vi "Omniax_mDrive_Zonly_2017APXNoBK_202107bk.vi"() -> ()   [LabVIEW 2015]
uses:
  <vilib>/Utility/file.llb/Read From Spreadsheet File (I64).vi
  <vilib>/Utility/file.llb/Read From Spreadsheet File (string).vi
  <userlib>/caLab/Private/Put_DBL_PV.vi
  <vilib>/Instr/_visa.llb/VISA Configure Serial Port (Instr).vi
  <userlib>/caLab/Private/Put_DBL-1D_PV-1D.vi
  <userlib>/caLab/Private/Get_PV.vi
  <userlib>/caLab/Private/Put_I16-1D_PV-1D.vi
  <userlib>/caLab/Private/Get_PV-1D.vi
  <vilib>/Utility/file.llb/Write To Spreadsheet File (I64).vi
panel:
  out "Status Message 2":string="HP cell pressure too high! or "
  out "APX:MZ_STOP":bool
  out "inside IV5?":bool
  out "APX:MZ_LIM-":bool
  out "inside PRP?":bool
  out "error out 2":errorcluster caption="error out"
  out "APX:MZ_CHK":u32
  out "APX:MZ_STAT":u32
  out "retracted":bool
  out "facingup":bool
  out "gatevalve":bool
  in  "Local":bool
  out "unsigned 8bit integer":u8
  out "SES is not busy":bool
  out "EPICS RQs":dbl[][](array[numeric])
  out "Status":bool
  in  "Pressure Overide":bool
  in  "Crash Override":bool
  in  "Is the gatevalve opened?\nAPX:MZ_CHK0":bool
  in  "Is the sample facinng up?\nAPX:MZ_CHK1":bool
  in  "Is the source retracted?\nAPX:MZ_CHK2":bool
  out "APX:MZ_MVG":bool
  out "inside HPC?":bool
  out "HPC01<0.001?":bool
  out "APX:V5 opened?":bool
  out "Isolated from GND?":bool
  out "APX:MZ_LIM+":bool
  out "APX:MZ_RDY":bool
  in  "APX:MZ_RQ":dbl=10.0 min=10.0 max=60.0 step=0.1 format="%_6g"
  in  "APX:MZ_VLC_RQ":dbl=0.40000000000000013 min=0.1 max=0.61 step=0.1
  out "Z Velocity SP step/sec":i32=102400 min=1 max=153600
  out "Z Step SP":i32=-20000 min=0 max=102400000 step=500
  out "Z Step PV":i32 max=2000
  out "Dev1AI0 Voltage":dbl
  out "Z max step":i32
  in  "V5 position 15360000":i32
  out "APX:MZ_VLC_PV":dbl format="%.3f"
  out "Presets":i32[][](array[numeric])
  in  "stop":bool
  in  "Tab Control 3":enum32{"Console", "Reset", "Bypass"}(tab)
  out "APX:MZ status":string="Cancel"
  out "Status Message":string="HP cell pressure too high! or "
  in  "Reset Z Position mm":dbl
  out "Reset Z Motor Steps":i32
  in  "Reset":bool
  out "Z Position MV mm":dbl
  in  "Clear ZY":bool
  out "R Backlash steps/sec":i32
  out "R Backlash":i32
  out "R Holding Current %":i32
  out "R Run Current %":i32
  out "R offset deg":dbl
  out "R deg/rev":dbl
  out "R steps/rev":u32
  out "R velocity PV step/sec":i32
  out "Z COM PORT":refnum<visa-resource-name>="COM5"
  out "Z Backlash steps/sec":i32
  out "Z Backlash":i32
  out "Z Holding Current %":i32
  out "Z Run Current %":i32
  out "Z offset mm":dbl
  out "Z mm/rev":dbl
  out "Z steps/rev":u32
  out "Z  velocity PV step/sec":i32=102400
  out "Z MINPOS":i32=-94296
  out "Z MAXPOS":i32=-34296
  out "APX:MZ_PV":dbl format="%_5g"
  out "X velocity PV step/sec":i32
  out "X Backlash steps/sec":i32
  out "X Backlash":i32
  out "X Holding Current %":i32
  out "X Run Current %":i32
  out "X offset mm":dbl
  out "X mm/rev":dbl
  out "X steps/rev":u32
  out "Y Backlash steps/sec":i32
  out "Y Backlash":i32
  out "Y Holding Current %":i32
  out "Y Run Current %":i32
  out "Y offset mm":dbl
  out "Y mm/rev":dbl
  out "Y steps/rev":u32
  out "Y velocity PV step/sec":i32
  in  "APX:MZ_STOP_Button":bool
  # "APX:MZ"
  # "v2022.06"
  # "COM14"
  # "Prep to Main checkpoints"
  # "Disable these"
  # "355.7"
  # "20 degree"
  # "290"
  # "60"
  # "355.7"
  # "10"
  # "289"
  # "55"
types:
  T1 = enum16{"Stop", "Reset", "Run Current", "Holding Current", "Accel Rate", "Decel Rate", "Move to Relative Position", "Move to Absolute Position", "Echo Mode", "Print Parameter", "Send String", "Microstep Resolution", "Set Current Position", "Max Velocity"}
  T2 = enum8{"Enabled", "Disabled", "Disabled and Grayed Out"}
  T3 = cluster{"first row[0]":i64, "first row[1]":i64, "first row[2]":i64, "first row[3]":i64, "first row[4]":i64, "first row[5]":i64, "first row[6]":i64, "first row[7]":i64, "first row[8]":i64}
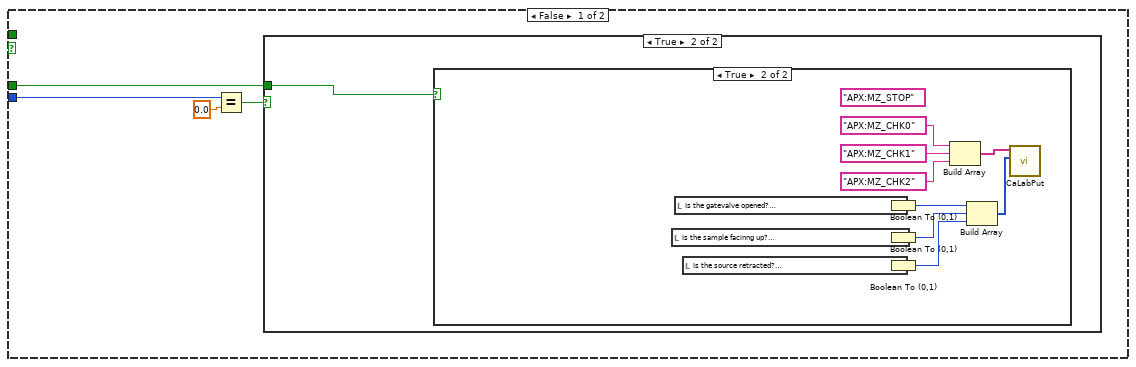
[diagram p3: hidden frame]
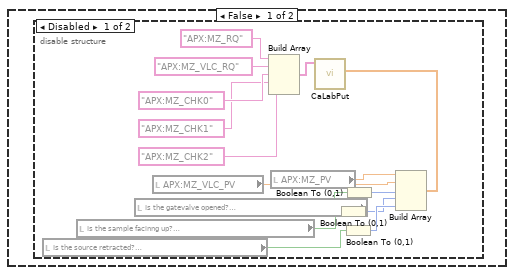
[diagram p5: hidden frame]
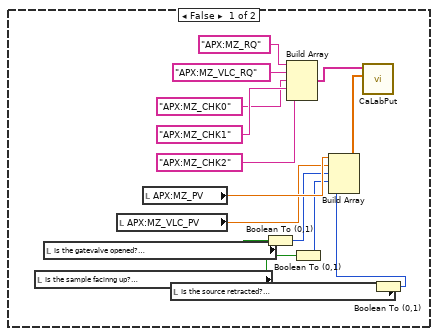
[diagram p7: hidden frame]
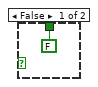
[diagram p10: hidden frame]
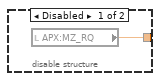
[diagram p12: hidden frame]
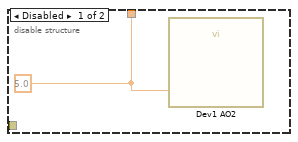
[diagram p14: hidden frame]
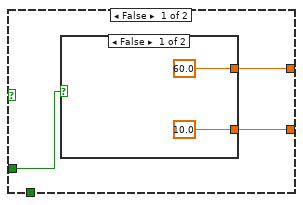
[diagram p16: hidden frame]
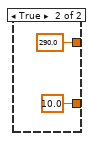
[diagram p17: hidden frame]
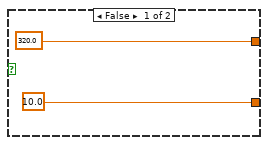
[diagram p18: hidden frame]
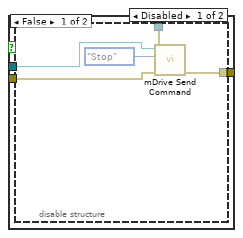
[diagram p19: hidden frame]
diagram:
  w4 = 0 ("dimension size")
  (unwired) 6144000 ("upper limit")
  (unwired) -6144000 ("lower limit")
  n1 = flat-sequence {
    tunnel: [w41] -> w23
    tunnel: [w42] -> w22
    tunnel: w23 -> [w57]
    tunnel: w22 -> [w56]
    tunnel: [w54] -> w2
    tunnel: [w52] -> w1
    tunnel: [w64] -> w27
    tunnel: [w60] -> w26
    tunnel: w2 -> [w61]
    tunnel: w1 -> [w60]
    tunnel: [w71] -> w38
    tunnel: [w73] -> w37
    tunnel: w27 -> [w72]
    tunnel: w26 -> [w74]
    tunnel: w38 -> [w81]
    tunnel: [w80] -> w36
    tunnel: w37 -> [w78]
    tunnel: [w79] -> w35
    tunnel: [w92] -> w34
    tunnel: [w93] -> w33
    tunnel: w36 -> [w91]
    tunnel: w35 -> [w90]
    tunnel: w34 -> [w103]
    tunnel: w33 -> [w102]
    tunnel: [w105] -> w32
    tunnel: [w104] -> w31
    tunnel: [w99] -> w30
    tunnel: [w112] -> w28
    tunnel: [w113] -> w29
    tunnel: w32 -> [w113]
    tunnel: w31 -> [w112]
    tunnel: w30 -> [w110]
    frame #0 {
      n2 = call-poly <userlib>:"CaLabPut.vi"("Value"=1.0, "PV Name"="SES:CalOff_RQ") -> ()  [unwired: 6 in, 4 out]
    }
    frame #1 {
      w49 = refnum<visa-resource-name> "COM14" ("COM PORT")
      w47 = u16 0 items=["None", "XON/XOFF", "RTS/CTS", "XON/XOFF & RTS/CTS", "DTR/DSR", "XON/XOFF & DTR/DSR"] ("flow control (0:none)")
      w46 = u16 10 items=["1.0"=10, "1.5"=15, "2.0"=20] ("stop bits (10: 1 bit)")
      # "Stop bits"
      n3 = call-poly "VISA Configure Serial Port"("VISA resource name"=w49, "timeout (10sec)"=u32 10000, "baud rate (9600)"=u32 9600, "data bits (8)"=u16 8, "parity (0:none)"=enum16{"None", "Odd", "Even", "Mark", "Space"}."None", "stop bits (10: 1 bit)"=w46, "flow control (0:none)"=w47) -> ("VISA resource name out"=w41:refnum<visa-resource-name>, "error out"=w42:errorcluster)  [unwired: 7 in]
      "Z COM PORT" <- w49
    }
    frame #2 {
      n4 = call "mDrive Send Command.vi"("error in (no error)"=w56, "Extra"="EM 2", "Command"=T1."Send String", "VISA resource name"=w57) -> ("error out"=w53:errorcluster, "VISA resource name out"=w55:refnum<visa-resource-name>)  [unwired: 3 in, 1 out]
      n5 = call "mDrive Send Command.vi"("error in (no error)"=w53, "Extra"="PR EE", "Command"=T1."Send String", "VISA resource name"=w55) -> ("error out"=w52:errorcluster, "VISA resource name out"=w54:refnum<visa-resource-name>)  [unwired: 3 in, 1 out]
    }
    frame #3 {
      n6 = Number To Decimal String(number=1000000) -> (decimal integer string=w62:string)  [unwired: 1 in]
      n7 = call "mDrive Send Command.vi"("Extra"=w62, "Command"=T1."Accel Rate", "VISA resource name"=w61) -> ("VISA resource name out"=w67:refnum<visa-resource-name>)  [unwired: 4 in, 2 out]
      n8 = call "mDrive Send Command.vi"("Extra"=w62, "Command"=T1."Decel Rate", "VISA resource name"=w67) -> ("VISA resource name out"=w64:refnum<visa-resource-name>)  [unwired: 4 in, 2 out]
    }
    frame #4 {
      # "Run Current %"
      n9 = property on="Z Run Current %" class="DigNum (strict)"() -> ("Value"=w69:i32)  [unwired: 2 in, 2 out]
      n10 = Number To Decimal String(number=w69) -> (decimal integer string=w70:string)  [unwired: 1 in]
      n11 = call "mDrive Send Command.vi"("error in (no error)"=w74, "Extra"=w70, "Command"=T1."Run Current", "VISA resource name"=w72) -> ("error out"=w73:errorcluster, "VISA resource name out"=w71:refnum<visa-resource-name>)  [unwired: 3 in, 1 out]
    }
    frame #5 {
      # "Holding Current %"
      n12 = property on="Z Run Current %" class="DigNum (strict)"() -> ("Value"=w76:i32)  [unwired: 2 in, 2 out]
      n13 = Number To Decimal String(number=w76) -> (decimal integer string=w77:string)  [unwired: 1 in]
      n14 = call "mDrive Send Command.vi"("error in (no error)"=w78, "Extra"=w77, "Command"=T1."Holding Current", "VISA resource name"=w81) -> ("error out"=w79:errorcluster, "VISA resource name out"=w80:refnum<visa-resource-name>)  [unwired: 3 in, 1 out]
    }
    frame #6 {
      # "Velocity Max"
      n15 = property on="Z Velocity SP step/sec" class="DigNum (strict)"() -> ("Value"=w89:i32)  [unwired: 2 in, 2 out]
      n16 = Number To Decimal String(number=w89) -> (decimal integer string=w88:string)  [unwired: 1 in]
      n17 = call "mDrive Send Command.vi"("error in (no error)"=w90, "Extra"=w88, "Command"=T1."Max Velocity", "VISA resource name"=w91) -> ("error out"=w86:errorcluster, "VISA resource name out"=w96:refnum<visa-resource-name>)  [unwired: 3 in, 1 out]
      n18 = call "mDrive Send Command.vi"("error in (no error)"=w86, "Extra"="VM", "Command"=T1."Print Parameter", "VISA resource name"=w96) -> ("error out"=w93:errorcluster, "read buffer"=w94:string, "VISA resource name out"=w92:refnum<visa-resource-name>)  [unwired: 3 in]
      n19 = Decimal String To Number(string=w94, offset=0) -> (number=w87:i32)  [unwired: 1 in, 1 out]
      n20 = local write "Local"(FALSE ("Remote")) -> ()
      n21 = property on="Z  velocity PV step/sec" class="DigNum (strict)"("Val(Sgnl)"=w87) -> ()  [unwired: 2 in, 2 out]
    }
    frame #7 {
      # "PRINT POSITION"
      n22 = call "mDrive Send Command.vi"("error in (no error)"=w102, "Extra"="P", "Command"=T1."Print Parameter", "VISA resource name"=w103) -> ("error out"=w104:errorcluster, "read buffer"=w101:string, "VISA resource name out"=w105:refnum<visa-resource-name>)  [unwired: 3 in]
      n23 = Decimal String To Number(string=w101, offset=0) -> (number=w99:i32)  [unwired: 1 in, 1 out]
    }
    frame #8 {
      n24 = property on="Z Step SP" class="DigNum (strict)"("Val(Sgnl)"=w110) -> ()  [unwired: 2 in, 2 out]
      n25 = property on="Z Step SP" class="DigNum (strict)"() -> ("Maximum"=w107:dbl)  [unwired: 2 in, 2 out]
      n26 = property on="Z Step SP" class="DigNum (strict)"() -> ("Minimum"=w109:dbl)  [unwired: 2 in, 2 out]
      n27 = To Long Integer(number=w107) -> (32bit integer=w108:i32)
      "Z MAXPOS" <- w108
      n28 = To Long Integer(number=w109) -> (32bit integer=w106:i32)
      "Z MINPOS" <- w106
      n29 = In Range and Coerce(upper limit=w108, x=w110, lower limit=w106) -> (In Range?=w111:bool)  [unwired: 1 out]
      n30 = property on="APX:MZ_LIM+" class="Bool (strict)"("Val(Sgnl)"=w111) -> ()  [unwired: 2 in, 2 out]
    }
  }
  n31 = flat-sequence {
    frame #0 {
      (unwired) 1.0 ("Data Entry Limits:Minimum")
      w117 = -3.0 ("R deg/rev")
      w115 = u32 51200 ("step/rev")
      n32 = To Double Precision Float(number=w115) -> (double precision float=w116:dbl)
      n33 = To Double Precision Float(number=10000 ("Value (Signaling)")) -> (double precision float=w121:dbl)
      n34 = Divide(x=w121, y=w116) -> (x/y=w120:dbl)
      n35 = Multiply(x=w120, y=w117) -> (x*y=w118:dbl)
      n36 = Absolute Value(x=w118) -> ()  [unwired: 1 out]
      "R offset deg" <- 0.0 ("R offset deg")
      "R deg/rev" <- w117
      "R steps/rev" <- w115
    }
  }
  n37 = flat-sequence {
    frame #0 {
      w124 = 0.2 ("Z mm/rev")
      w123 = u32 51200 ("step/rev")
      n38 = To Double Precision Float(number=153600 ("Value (Signaling)")) -> (double precision float=w129:dbl)
      n39 = To Double Precision Float(number=w123) -> (double precision float=w128:dbl)
      n40 = property on="Z Velocity SP step/sec" class="DigNum (strict)"("Val(Sgnl)"=51200 ("Value (Signaling)")) -> ()  [unwired: 2 in, 2 out]
      n41 = property on="Z Velocity SP step/sec" class="DigNum (strict)"("Minimum"=1.0 ("Data Entry Limits:Minimum")) -> ()  [unwired: 2 in, 2 out]
      n42 = Divide(x=w129, y=w128) -> (x/y=w126:dbl)
      n43 = property on="Z Velocity SP step/sec" class="DigNum (strict)"("Maximum"=w129) -> ()  [unwired: 2 in, 2 out]
      n44 = Multiply(x=w126, y=w124) -> (x*y=w127:dbl)
      n45 = property on="APX:MZ_VLC_RQ" class="DigNum (strict)"("Val(Sgnl)"=w127) -> ()  [unwired: 2 in, 2 out]
      "Z offset mm" <- 0.0 ("Z offset mm")
      "Z mm/rev" <- w124
      "Z steps/rev" <- w123
    }
  }
  n46 = disable-structure shown="Disabled" {
    frame Disabled {
      n47 = flat-sequence {
        frame #0 {
          w132 = FALSE ("Value (Signaling)")
          w135 = FALSE ("Value (Signaling)")
          w138 = FALSE ("Value (Signaling)")
          w139 = FALSE ("Value (Signaling)")
          "Z Backlash steps/sec" <- 25600 ("Z Backlash steps/sec")
          "Z Backlash" <- -51200 ("Z Backlash")
          "X Backlash steps/sec" <- 25600 ("Value (Signaling)")
          "X Backlash" <- 10240 ("Backlash2")
          "Y Backlash" <- -10240 ("Backlash2")
          "Y Backlash steps/sec" <- 25600 ("Value (Signaling)")
          "R Backlash steps/sec" <- 6400 ("R Backlash steps/sec")
          "R Backlash" <- -12800 ("R Backlash")
        }
      }
    }
    frame Enabled {
    }
  }
  n48 = flat-sequence {
    frame #0 {
      "Z Holding Current %" <- 20 ("Z Holding Current %")
      "Z Run Current %" <- 40 ("Z Run Current %")
      "X Run Current %" <- 40 ("Run Current %")
      "X Holding Current %" <- 20 ("Holding Current %")
      "Y Run Current %" <- 40 ("Run Current %")
      "Y Holding Current %" <- 20 ("Holding Current %")
      "R Holding Current %" <- 15 ("R Holding Current %")
      "R Run Current %" <- 80 ("R Run Current %")
    }
  }
  n49 = flat-sequence {
    frame #0 {
      (unwired) 0.1 ("Value (Signaling)")
      (unwired) FALSE ("Value (Signaling)")
      (unwired) T2."Disabled and Grayed Out" ("Disabled")
      (unwired) T2."Disabled and Grayed Out" ("Disabled")
      (unwired) 0.1 ("Value (Signaling)")
      (unwired) FALSE ("Value (Signaling)")
      (unwired) 0.1 ("Value (Signaling)")
      (unwired) FALSE ("Value (Signaling)")
      (unwired) 0.1 ("Value (Signaling)")
      (unwired) FALSE ("Value (Signaling)")
    }
  }
  n50 = flat-sequence {
    frame #0 {
      w154 = 0.2 ("MM/rev")
      w156 = u32 51200 ("step/rev")
      (unwired) 1.0 ("Data Entry Limits:Minimum")
      # "a=1000000"
      n51 = To Double Precision Float(number=128000 ("Value (Signaling)")) -> (double precision float=w157:dbl)
      n52 = To Double Precision Float(number=w156) -> (double precision float=w155:dbl)
      n53 = Divide(x=w157, y=w155) -> (x/y=w153:dbl)
      n54 = Multiply(x=w153, y=w154) -> ()  [unwired: 1 out]
      "X offset mm" <- 0.0 ("offset")
      "X steps/rev" <- w156
      "X mm/rev" <- w154
    }
  }
  n55 = flat-sequence {
    frame #0 {
      w161 = 0.2 ("MM/rev")
      w163 = u32 51200 ("step/rev")
      (unwired) 1.0 ("Data Entry Limits:Minimum")
      n56 = To Double Precision Float(number=128000 ("Value (Signaling)")) -> (double precision float=w164:dbl)
      n57 = To Double Precision Float(number=w163) -> (double precision float=w162:dbl)
      n58 = Divide(x=w164, y=w162) -> (x/y=w160:dbl)
      n59 = Multiply(x=w160, y=w161) -> ()  [unwired: 1 out]
      "Y offset mm" <- 0.0 ("offset")
      "Y steps/rev" <- w163
      "Y mm/rev" <- w161
    }
  }
  n60 = property on="Z Step SP" class="DigNum (strict)"("Minimum"=0 ("lower limit")) -> ()  [unwired: 2 in, 2 out]
  n61 = property on="V5 position 15360000" class="DigNum (strict)"("Value"=15360000 ("V5 position 15360000")) -> ()  [unwired: 2 in, 2 out]
  n62 = property on="Z Step SP" class="DigNum (strict)"("Maximum"=102400000 ("upper limit")) -> ()  [unwired: 2 in, 2 out]
  n63 = call-poly <vilib>:"Read From Spreadsheet File.vi"("file path (dialog if empty)"=path "T:/PAR/IMS/POSZ.TXT") -> ("first row"=w18:i64[])  [unwired: 6 in, 4 out]
  n64 = call-poly <vilib>:"Read From Spreadsheet File.vi"("file path (dialog if empty)"=path "T:/PAR/IMS/PRESET.TXT") -> ("all rows"=w10:string[][])  [unwired: 6 in, 4 out]
  n65 = Array To Cluster(array=w18) -> (cluster=w17:T3)
  n66 = Transpose 2D Array(2D array=w10) -> (transposed array=w11:string[][])
  n67 = Unbundle(w17) -> ("first row[2]"=w15:i64)  [unwired: 8 out]
  n68 = Delete From Array(array=w11, index (row)=0) -> (array with subset deleted=w13:string[][])  [unwired: 2 in, 1 out]
  n69 = property on="Reset Z Motor Steps" class="DigNum (strict)"("Val(Sgnl)"=w15) -> ()  [unwired: 2 in, 2 out]
  n70 = Transpose 2D Array(2D array=w13) -> (transposed array=w14:string[][])
  n71 = Decimal String To Number(string=w14) -> (number=w12:i32[][])  [unwired: 2 in, 1 out]
  n72 = Initialize Array(w4, w4, 4 ("dimension size")) -> (w7:i32[][])
  n73 = Build Array (concatenate)(w7, w12) -> (→"Presets":i32[][])
  n74 = while {
    tunnel: w29 -> [w181]
    tunnel: w28 -> [w180]
    tunnel: [w179] -> w21
    tunnel: [w178] -> w20
    tunnel: [w177] -> _
    tunnel: [w176] -> _
    i -> [w168]
    stop <- "stop" stop-if-true
    n75 = flat-sequence {
      frame #0 {
        (unwired) 0
        (unwired) "APX:MZ_STOP"
        n76 = local read "Is the gatevalve opened?\nAPX:MZ_CHK0"() -> (w203:bool)
        n77 = local read "Is the source retracted?\nAPX:MZ_CHK2"() -> (w205:bool)
        n78 = local read "Is the sample facinng up?\nAPX:MZ_CHK1"() -> (w204:bool)
        n79 = local read "SES is not busy"() -> (w189:bool)
        n80 = local read "APX:MZ_LIM+"() -> (w194:bool)
        n81 = local read "APX:MZ_RDY"() -> (w196:bool)
        n82 = local read "APX:MZ_MVG"() -> (w195:bool)
        n83 = local read "APX:MZ_LIM-"() -> (w193:bool)
        n84 = local read "Isolated from GND?"() -> (w192:bool)
        n85 = local read "inside HPC?"() -> (w190:bool)
        n86 = local read "HPC01<0.001?"() -> (w188:bool)
        n87 = local read "APX:V5 opened?"() -> (w191:bool)
        n88 = local read "inside PRP?"() -> (w186:bool)
        n89 = local read "inside IV5?"() -> (w185:bool)
        n90 = local read "Dev1AI0 Voltage"() -> (w183:dbl)
        n91 = Build Array(w196, w195, w194, w193, w192, w191, w186, w185, w190, w189, w188) -> (w187:bool[])
        n92 = Build Array(w203, w204, w205) -> (w206:bool[])
        n93 = Boolean Array To Number(Boolean array=w187) -> (number=w199:u32)
        "APX:MZ_STAT" <- w199
        n94 = Boolean Array To Number(Boolean array=w206) -> (number=w200:u32)
        "APX:MZ_CHK" <- w200
        n95 = Build Array(w200, w199, w183) -> (w197:dbl[])
        n96 = Build Array("APX:MZ_CHK", "APX:MZ_STAT", "SSE:Tsample") -> (w198:string[])
        n97 = call-poly <userlib>:"CaLabPut.vi"("Values"=w197, "PV Names"=w198) -> ()  [unwired: 6 in, 4 out]
      }
    }
    n98 = Quotient & Remainder(x=w168, y=2) -> (x-y*floor(x/y)=w173:i32)  [unwired: 1 out]
    n99 = Greater?(x=w168, y=2.0) -> (0:w169:bool)
    n100 = Equal To 0?(x=w173) -> (x = 0?=w174:bool)
    n101 = case shown="True" w174 {
      tunnel: [FALSE ("Status") TRUE ("Status")] -> w171
      frame False {
      }
      frame True {
      }
    }
    n102 = Not(x="Local") -> (.not. x?=w166:bool)
    n103 = case shown="True" w169 {
      tunnel: w171 -> [_ w239]
      tunnel: w168 -> [w209 _]
      tunnel: w166 -> [w207 w238]
      frame False {
        n104 = Equal?(x=w209, y=0.0) -> (x = y?=w208:bool)
        n105 = case shown="True" w208 {
          tunnel: w207 -> [_ w211]
          frame False {
          }
          frame True {
            n106 = case shown="True" w211 {
              frame False {
                n107 = disable-structure shown="Disabled" {
                  frame Disabled {
                    n108 = local read "Is the source retracted?\nAPX:MZ_CHK2"() -> (w212:bool)
                    n109 = local read "Is the sample facinng up?\nAPX:MZ_CHK1"() -> (w213:bool)
                    n110 = local read "Is the gatevalve opened?\nAPX:MZ_CHK0"() -> (w214:bool)
                    n111 = local read "APX:MZ_VLC_PV"() -> (w221:dbl)
                    n112 = Build Array("APX:MZ_RQ", "APX:MZ_VLC_RQ", "APX:MZ_CHK0", "APX:MZ_CHK1", "APX:MZ_CHK2") -> (w224:string[])
                    n113 = local read "APX:MZ_PV"() -> (w222:dbl)
                    n114 = Boolean To (0,1)(Boolean=w213) -> (0, 1=w215:i16)
                    n115 = Boolean To (0,1)(Boolean=w212) -> (0, 1=w217:i16)
                    n116 = Boolean To (0,1)(Boolean=w214) -> (0, 1=w216:i16)
                    n117 = Build Array(w222, w221, w216, w215, w217) -> (w223:dbl[])
                    n118 = call-poly <userlib>:"CaLabPut.vi"("Values"=w223, "PV Names"=w224) -> ()  [unwired: 6 in, 4 out]
                  }
                  frame Enabled {
                  }
                }
              }
              frame True {
                (unwired) "APX:MZ_STOP"
                n119 = local read "Is the sample facinng up?\nAPX:MZ_CHK1"() -> (w232:bool)
                n120 = local read "Is the gatevalve opened?\nAPX:MZ_CHK0"() -> (w233:bool)
                n121 = local read "Is the source retracted?\nAPX:MZ_CHK2"() -> (w231:bool)
                n122 = Boolean To (0,1)(Boolean=w233) -> (0, 1=w230:i16)
                n123 = Boolean To (0,1)(Boolean=w232) -> (0, 1=w229:i16)
                n124 = Boolean To (0,1)(Boolean=w231) -> (0, 1=w228:i16)
                n125 = Build Array("APX:MZ_CHK0", "APX:MZ_CHK1", "APX:MZ_CHK2") -> (w234:string[])
                n126 = Build Array(w230, w229, w228) -> (w227:i16[])
                n127 = call-poly <userlib>:"CaLabPut.vi"("Values"=w227, "PV Names"=w234) -> ()  [unwired: 6 in, 4 out]
              }
            }
          }
        }
      }
      frame True {
        n128 = case shown="True" w238 {
          frame False {
            n129 = local read "Is the sample facinng up?\nAPX:MZ_CHK1"() -> (w245:bool)
            n130 = local read "Is the gatevalve opened?\nAPX:MZ_CHK0"() -> (w246:bool)
            n131 = local read "APX:MZ_VLC_PV"() -> (w247:dbl)
            n132 = local read "APX:MZ_PV"() -> (w248:dbl)
            n133 = local read "Is the source retracted?\nAPX:MZ_CHK2"() -> (w244:bool)
            n134 = Boolean To (0,1)(Boolean=w246) -> (0, 1=w243:i16)
            n135 = Build Array("APX:MZ_RQ", "APX:MZ_VLC_RQ", "APX:MZ_CHK0", "APX:MZ_CHK1", "APX:MZ_CHK2") -> (w251:string[])
            n136 = Boolean To (0,1)(Boolean=w245) -> (0, 1=w242:i16)
            n137 = Boolean To (0,1)(Boolean=w244) -> (0, 1=w241:i16)
            n138 = Build Array(w248, w247, w243, w242, w241) -> (w240:dbl[])
            n139 = call-poly <userlib>:"CaLabPut.vi"("Values"=w240, "PV Names"=w251) -> ()  [unwired: 6 in, 4 out]
          }
          frame True {
            w273 = 0 ("index (col)")
            n140 = Build Array("APX:MZ_RQ", "APX:MZ_VLC_RQ", "APX:MZ_STOP", "APX:MZ_CHK0", "APX:MZ_CHK1", "APX:MZ_CHK2") -> (w301:string[])
            n141 = call-poly "CaLabGet.vi"("PV Names"=w301) -> ("Value Array (number)"=w272:dbl[][])  [unwired: 8 in, 6 out]
            "EPICS RQs" <- w272
            n142 = Index Array(array=w272, index (row)=0, index (col)=w273) -> (element=w293:dbl)
            n143 = Index Array(array=w272, index (row)=1, index (col)=w273) -> (element=w296:dbl)
            n144 = Index Array(array=w272, index (row)=2, index (col)=w273) -> (element=w285:dbl)
            n145 = Index Array(array=w272, index (row)=3, index (col)=w273) -> (element=w283:dbl)
            n146 = Index Array(array=w272, index (row)=4, index (col)=w273) -> (element=w270:dbl)
            n147 = Index Array(array=w272, index (row)=5, index (col)=w273) -> (element=w267:dbl)
            n148 = To Unsigned Byte Integer(number=w283) -> (unsigned 8bit integer=w282:u8)
            n149 = To Unsigned Byte Integer(number=w270) -> (unsigned 8bit integer=w271:u8)
            n150 = To Unsigned Byte Integer(number=w267) -> (unsigned 8bit integer=w268:u8)
            n151 = To Unsigned Byte Integer(number=w285) -> (unsigned 8bit integer=w265:u8)
            "unsigned 8bit integer" <- w265
            n152 = In Range and Coerce(upper limit=0.6, x=w296, lower limit=0.1) -> (coerced(x)=w289:dbl)  [unwired: 1 out]
            n153 = In Range and Coerce(upper limit=355.7, x=w293, lower limit=10.0) -> (coerced(x)=w290:dbl)  [unwired: 1 out]
            n154 = Number To Boolean Array(number=w282) -> (Boolean array=w276:bool[])
            n155 = Number To Boolean Array(number=w271) -> (Boolean array=w269:bool[])
            n156 = Number To Boolean Array(number=w268) -> (Boolean array=w266:bool[])
            n157 = Index Array(array=w276, index=0) -> (element=w258:bool)
            "gatevalve" <- w258
            n158 = Index Array(array=w269, index=0) -> (element=w259:bool)
            "facingup" <- w259
            n159 = Index Array(array=w266, index=0) -> (element=w260:bool)
            "retracted" <- w260
            n160 = Number To Boolean Array(number=w265) -> (Boolean array=w257:bool[])
            n161 = local write "Is the source retracted?\nAPX:MZ_CHK2"(w260) -> ()
            n162 = local read "APX:MZ_RQ"() -> (w264:dbl)
            n163 = local write "Is the gatevalve opened?\nAPX:MZ_CHK0"(w258) -> ()
            n164 = local read "APX:MZ_VLC_RQ"() -> (w263:dbl)
            n165 = Index Array(array=w257, index=0) -> (element=w255:bool)
            n166 = local write "Is the sample facinng up?\nAPX:MZ_CHK1"(w259) -> ()
            n167 = local write "APX:MZ_STOP"(w255) -> ()
            n168 = Equal?(x=w264, y=w290) -> (x = y?=w262:bool)
            n169 = Equal?(x=w263, y=w289) -> (x = y?=w261:bool)
            n170 = case shown="False" w262 {
              tunnel: w290 -> [w303 _]
              frame False {
                n171 = property on="APX:MZ_RQ" class="DigNum (strict)"("Val(Sgnl)"=w303) -> ()  [unwired: 2 in, 2 out]
              }
              frame True {
              }
            }
            n172 = case shown="False" w261 {
              tunnel: w289 -> [w302 _]
              frame False {
                n173 = property on="APX:MZ_VLC_RQ" class="DigNum (strict)"("Val(Sgnl)"=w302) -> ()  [unwired: 2 in, 2 out]
              }
              frame True {
              }
            }
          }
        }
        "Status" <- w239
      }
    }
    n174 = event shown="[0] Timeout" {
      selector: _ -> [_ _ _ _ _ _]
      dyn-events: _ -> [_ _ _ _ _ _]
      timeout: 100 -> [_ _ _ _ _ _]
      tunnel: w181 -> [w338 _ _ w662 w737 w746]
      tunnel: w180 -> [w339 _ _ w661 w736 w745]
      tunnel: [w353 _ _ w659 w735 _] -> w179
      tunnel: [w352 _ _ w660 w734 _] -> w178
      tunnel: [_ _ _ _ _ w744] -> w177
      tunnel: [_ _ _ _ _ w743] -> w176
      event Timeout {
        n175 = event-data() -> ()  [unwired: 1 in, 2 out]
        n176 = disable-structure shown="Disabled" {
          frame Disabled {
            n177 = property on="Local" class="Bool (strict)"() -> ("Value"=w365:bool)  [unwired: 2 in, 2 out]
            n178 = case shown="True" w365 {
              frame False {
              }
              frame True {
                n179 = disable-structure shown="Enabled" {
                  disable-tunnel: [w368 w369] -> w366
                  frame Disabled {
                    n180 = local read "APX:MZ_RQ"() -> (w368:dbl)
                  }
                  frame Enabled {
                    n181 = property on="APX:MZ_RQ" class="DigNum (strict)"() -> ("Value"=w369:dbl)  [unwired: 2 in, 2 out]
                  }
                }
                n182 = call-poly <userlib>:"CaLabPut.vi"("Value"=w366, "PV Name"="APX:MZ_RQ") -> ()  [unwired: 6 in, 4 out]
              }
            }
          }
          frame Enabled {
          }
        }
        n183 = property on="Is the gatevalve opened?\nAPX:MZ_CHK0" class="Bool (strict)"() -> ("Value"=w324:bool)  [unwired: 2 in, 2 out]
        n184 = property on="Is the sample facinng up?\nAPX:MZ_CHK1" class="Bool (strict)"() -> ("Value"=w325:bool)  [unwired: 2 in, 2 out]
        n185 = property on="Is the source retracted?\nAPX:MZ_CHK2" class="Bool (strict)"() -> ("Value"=w326:bool)  [unwired: 2 in, 2 out]
        n186 = property on="Isolated from GND?" class="Bool (strict)"() -> ("Value"=w343:bool)  [unwired: 2 in, 2 out]
        n187 = property on="Is the source retracted?\nAPX:MZ_CHK2" class="Bool (strict)"() -> ("Value"=w334:bool)  [unwired: 2 in, 2 out]
        n188 = And(x=w325, y=w326) -> (x .and. y?=w323:bool)
        n189 = And(x=w324, y=w323) -> (x .and. y?=w322:bool)
        n190 = flat-sequence {
          tunnel: [w413] -> w335
          frame #0 {
            n191 = case shown="False" "Pressure Overide" {
              tunnel: [w415 TRUE] -> w413
              frame False {
                n192 = call-poly "CaLabGet.vi"("PV Name"="APX:HPC01") -> ("1rst Value (number)"=w430:dbl, "Error out"=w427:errorcluster)  [unwired: 8 in, 5 out]
                n193 = call-poly "CaLabGet.vi"("PV Name"="APX:V5_SOP", "Error in (no error)"=w427) -> ("1rst Value (number)"=w426:dbl, "Error out"=w419:errorcluster)  [unwired: 7 in, 5 out]
                n194 = call-poly "CaLabGet.vi"("PV Name"="SES:BUSY", "Error in (no error)"=w419) -> ("1rst Value (number)"=w418:dbl)  [unwired: 7 in, 6 out]
                n195 = Less?(x=w430, y=0.001) -> (x < y?=w424:bool)
                "HPC01<0.001?" <- w424
                n196 = Equal?(x=w418, y=0.0) -> (x = y?=w414:bool)
                "SES is not busy" <- w414
                n197 = Number To Boolean Array(number=w426) -> (Boolean array=w425:bool[])
                n198 = case shown="True" w424 {
                  tunnel: ["HP cell pressure too high!" w435] -> w423
                  frame False {
                  }
                  frame True {
                    n199 = local read "Status Message"() -> (w435:string)
                  }
                }
                n200 = Index Array(array=w425) -> (element=w421:bool)  [unwired: 1 in]
                "APX:V5 opened?" <- w421
                n201 = case shown="False" w421 {
                  tunnel: ["HP Turbo GV is closed." w433] -> w422
                  frame False {
                  }
                  frame True {
                    n202 = local read "Status Message"() -> (w433:string)
                  }
                }
                n203 = Or(x=w424, y=w421) -> (x .or. y?=w416:bool)
                n204 = Or(x=w416, y=w414) -> (x .or. y?=w415:bool)
                n205 = local write "Status Message"(w423) -> ()
                n206 = local write "Status Message"(w422) -> ()
              }
              frame True {
              }
            }
          }
        }
        n207 = property on="Is the sample facinng up?\nAPX:MZ_CHK1" class="Bool (strict)"() -> ("Value"=w333:bool)  [unwired: 2 in, 2 out]
        n208 = case shown="True" w322 {
          tunnel: [w500 w501] -> w351
          frame False {
            n209 = property on="V5 position 15360000" class="DigNum (strict)"() -> ("Value"=w500:i32)  [unwired: 2 in, 2 out]
          }
          frame True {
            n210 = property on="Z Step SP" class="DigNum (strict)"() -> ("Maximum"=w501:dbl)  [unwired: 2 in, 2 out]
          }
        }
        "Z max step" <- w351
        n211 = local read "APX:MZ_VLC_PV"() -> (w317:dbl)
        n212 = Build Array("APX:MZ_PV" ("PV Name"), "APX:MZ_VLC_PV" ("PV Name")) -> (w314:string[])
        n213 = property on="Is the gatevalve opened?\nAPX:MZ_CHK0" class="Bool (strict)"() -> ("Value"=w340:bool)  [unwired: 2 in, 2 out]
        n214 = And(x=w333, y=w334) -> (x .and. y?=w332:bool)
        n215 = property on="APX:MZ_PV" class="DigNum (strict)"() -> ("Value"=w316:dbl)  [unwired: 2 in, 2 out]
        n216 = Build Array(w316, w317) -> (w315:dbl[])
        n217 = And(x=w340, y=w332) -> (x .and. y?=w346:bool)
        n218 = property on="inside HPC?" class="Bool (strict)"() -> ("Value"=w341:bool)  [unwired: 2 in, 2 out]
        n219 = call-poly <userlib>:"CaLabPut.vi"("Values"=w315, "PV Names"=w314) -> ()  [unwired: 6 in, 4 out]
        n220 = Greater Or Equal?(x=w316, y=320.0) -> (x >= y?=w327:bool)
        n221 = And(x=w343, y=w346) -> (x .and. y?=w321:bool)
        n222 = Greater?(x=w316, y=55.0) -> (0:w347:bool)
        n223 = Greater?(x=w316, y=289.0) -> (0:w331:bool)
        n224 = flat-sequence {
          frame #0 {
            w371 = 5 ("number of samples")
            # "ai16 p0.16"
            # "Crash Sensing"
            n225 = call "Dev1 AI0"("number of samples"=w371) -> ("data"=w376:dynamicdata, "error out"=w370:errorcluster)  [unwired: 16 in, 1 out]
            n226 = call "Convert from Dynamic Data"("Dynamic Data Type"=w376) -> ("Array"=w377:dbl[])  [unwired: 3 in]
            n227 = disable-structure shown="Enabled" {
              disable-tunnel: [w383 5.0 ("data")] -> w382
              disable-tunnel: w370 -> [_ w385]
              frame Disabled {
                w383 = 5.0 ("data")
                n228 = call "Dev1 AO2"("data"=w383) -> ()  [unwired: 17 in, 2 out]
              }
              frame Enabled {
                n229 = call "Dev1 P1.7"("data"=bool[] [TRUE], "error in"=w385) -> ("error out"=→"error out 2":errorcluster)  [unwired: 16 in, 1 out]
              }
            }
            n230 = Add Array Elements(numeric array=w377) -> (sum=w375:dbl)
            n231 = Divide(x=w375, y=w371) -> (x/y=w374:dbl)
            n232 = Absolute Value(x=w374) -> (abs(x)=w378:dbl)
            "Dev1AI0 Voltage" <- w378
            n233 = Multiply(x=w382, y=0.8) -> (x*y=w372:dbl)
            n234 = Greater?(x=w378, y=w372) -> (0:w379:bool)
            n235 = case shown="True" "Crash Override" {
              tunnel: [w388 TRUE] -> w380
              tunnel: w379 -> [w388 _]
              frame False {
              }
              frame True {
              }
            }
            "Isolated from GND?" <- w380
          }
        }
        n236 = case shown="False" w347 {
          tunnel: w343 -> [w447 _]
          tunnel: [w447 w455] -> w336
          tunnel: w321 -> [_ w455]
          tunnel: ["Sample is grounded!" w453] -> w344
          tunnel: w331 -> [_ w454]
          tunnel: w341 -> [_ w452]
          tunnel: w340 -> [_ w451]
          tunnel: w333 -> [_ w450]
          tunnel: [TRUE FALSE] -> w312
          tunnel: [FALSE TRUE] -> w311
          frame False {
            w438 = 0.0 ("element")
            w445 = FALSE ("Open?")
            n237 = Build Array("APX:MZ_CHK0" ("PV Name"), "APX:MZ_CHK1" ("PV Name"), "APX:MZ_CHK2" ("PV Name")) -> (w442:string[])
            n238 = property on="Is the gatevalve opened?\nAPX:MZ_CHK0" class="Bool (strict)"("Value"=w445) -> ()  [unwired: 2 in, 2 out]
            n239 = Build Array(w438, w438, w438) -> (w437:dbl[])
            n240 = property on="Is the source retracted?\nAPX:MZ_CHK2" class="Bool (strict)"("Value"=w445) -> ()  [unwired: 2 in, 2 out]
            n241 = property on="Is the sample facinng up?\nAPX:MZ_CHK1" class="Bool (strict)"("Value"=w445) -> ()  [unwired: 2 in, 2 out]
            n242 = call-poly <userlib>:"CaLabPut.vi"("Values"=w437, "PV Names"=w442) -> ()  [unwired: 6 in, 4 out]
          }
          frame True {
            n243 = case shown="False" w454 {
              tunnel: [w457 "Be careful, the sample enters into the HP cell!"] -> w453
              tunnel: w452 -> [_ _]
              tunnel: w451 -> [w462 _]
              tunnel: w450 -> [w461 _]
              frame False {
                w458 = "\r"
                w457 = "Is the gate valve opened? Is the sample facing up?  Is the lamp heater retracted?"
                n244 = disable-structure shown="Disabled" {
                  disable-tunnel: w462 -> [w467 _]
                  disable-tunnel: w461 -> [w466 _]
                  disable-tunnel: [w465 _] -> w460
                  disable-tunnel: [w464 _] -> w459
                  frame Disabled {
                    n245 = case shown="True" w467 {
                      tunnel: ["Is the sample facing up?" ""] -> w465
                      frame False {
                      }
                      frame True {
                      }
                    }
                    n246 = case shown="True" w466 {
                      tunnel: ["Is the gate valve opened?" ""] -> w464
                      frame False {
                      }
                      frame True {
                      }
                    }
                  }
                  frame Enabled {
                  }
                }
                n247 = property on="inside HPC?" class="Bool (strict)"("Value"=FALSE ("inside HPC?")) -> ()  [unwired: 2 in, 2 out]
                n248 = Concatenate Strings(w460, w458, w459, w458, w457) -> (w456:string)
                n249 = local write "Status Message"(w456) -> ()
              }
              frame True {
                w473 = 0.1 ("APX:MZ_VLC_RQ")
                n250 = property on="APX:MZ_VLC_RQ" class="DigNum (strict)"("Value"=w473) -> ()  [unwired: 2 in, 2 out]
                n251 = property on="inside HPC?" class="Bool (strict)"("Value"=TRUE ("inside HPC?")) -> ()  [unwired: 2 in, 2 out]
                n252 = call-poly <userlib>:"CaLabPut.vi"("Value"=w473, "PV Name"="APX:MZ_VLC_RQ") -> ()  [unwired: 6 in, 4 out]
                n253 = local write "Status Message 2"("Sample is touching HPC!") -> ()
              }
            }
          }
        }
        n254 = local write "inside PRP?"(w312) -> ()
        n255 = local write "inside IV5?"(w311) -> ()
        n256 = case shown="True" w335 {
          tunnel: w339 -> [w406 w411]
          tunnel: [w405 w411] -> w337
          tunnel: w338 -> [w404 _]
          frame False {
            n257 = disable-structure shown="Disabled" {
              disable-tunnel: w406 -> [w409 _]
              disable-tunnel: [w408 _] -> w405
              disable-tunnel: w404 -> [w407 _]
              frame Disabled {
                n258 = call "mDrive Send Command.vi"("error in (no error)"=w409, "Command"=T1."Stop", "VISA resource name"=w407) -> ("error out"=w408:errorcluster)  [unwired: 4 in, 2 out]
              }
              frame Enabled {
              }
            }
          }
          frame True {
          }
        }
        n259 = Or(x=w335, y=w336) -> (x .or. y?=w320:bool)
        n260 = property on="Isolated from GND?" class="Bool (strict)"() -> ("Value"=w319:bool)  [unwired: 2 in, 2 out]
        n261 = case shown="True" w331 {
          tunnel: [w392 w399] -> w330
          tunnel: [w391 w398] -> w329
          tunnel: w327 -> [_ w397]
          tunnel: w321 -> [w390 _]
          frame False {
            n262 = case shown="False" w390 {
              tunnel: [60.0 ("Data Entry Limits:Maximum") 290.0 ("Data Entry Limits:Maximum")] -> w392
              tunnel: [10.0 ("Data Entry Limits:Minimum") 10.0 ("Data Entry Limits:Minimum")] -> w391
              frame False {
              }
              frame True {
              }
            }
          }
          frame True {
            n263 = case shown="True" w397 {
              tunnel: [320.0 ("Data Entry Limits:Maximum") 355.7 ("Data Entry Limits:Maximum")] -> w399
              tunnel: [10.0 ("Data Entry Limits:Minimum") 290.0 ("Data Entry Limits:Minimum")] -> w398
              frame False {
              }
              frame True {
              }
            }
          }
        }
        n264 = And(x=w320, y=w319) -> (x .and. y?=w308:bool)
        n265 = local read "APX:MZ_STOP"() -> (w310:bool)
        n266 = Equal?(x=w310, y=FALSE) -> (x = y?=w307:bool)
        n267 = And(x=w308, y=w307) -> (x .and. y?=w306:bool)
        n268 = case shown="False" w306 {
          tunnel: w338 -> [w484 w497]
          tunnel: [w483 w497] -> w350
          tunnel: [w481 w494] -> w349
          tunnel: w344 -> [w480 _]
          tunnel: w343 -> [w479 _]
          tunnel: [w478 w496] -> w342
          tunnel: w341 -> [_ w495]
          tunnel: w337 -> [w477 w494]
          frame False {
            n269 = case shown="True" w479 {
              tunnel: w480 -> [w485 w487]
              tunnel: [w485 "Be careful!"] -> w478
              frame False {
              }
              frame True {
                n270 = disable-structure shown="Disabled" {
                  disable-tunnel: [w490 _] -> w488
                  disable-tunnel: w487 -> [w489 _]
                  frame Disabled {
                    n271 = Two Button Dialog(message=w489, 1:"Cancel" ("F button name (\"Cancel\")"), 2:"OK" ("T button name (\"OK\")")) -> (T button?=w490:bool)
                  }
                  frame Enabled {
                  }
                }
                n272 = disable-structure shown="Disabled" {
                  disable-tunnel: w488 -> [w493 _]
                  frame Disabled {
                    n273 = property on="Is the gatevalve opened?\nAPX:MZ_CHK0" class="Bool (strict)"("Value"=w493) -> ()  [unwired: 2 in, 2 out]
                    n274 = property on="inside HPC?" class="Bool (strict)"("Value"=w493) -> ()  [unwired: 2 in, 2 out]
                    n275 = property on="Is the sample facinng up?\nAPX:MZ_CHK1" class="Bool (strict)"("Value"=w493) -> ()  [unwired: 2 in, 2 out]
                  }
                  frame Enabled {
                  }
                }
              }
            }
            n276 = call "mDrive Send Command.vi"("error in (no error)"=w477, "Command"=T1."Stop", "VISA resource name"=w484) -> ("error out"=w481:errorcluster, "VISA resource name out"=w483:refnum<visa-resource-name>)  [unwired: 4 in, 1 out]
          }
          frame True {
            n277 = case shown="False" w495 {
              tunnel: ["Normal" "In HPC! Be careful! "] -> w496
              frame False {
              }
              frame True {
              }
            }
          }
        }
        "APX:MZ status" <- w342
        n278 = property on="APX:MZ_RQ" class="DigNum (strict)"("Maximum"=w330) -> ()  [unwired: 2 in, 2 out]
        n279 = property on="APX:MZ_RQ" class="DigNum (strict)"("Minimum"=w329) -> ()  [unwired: 2 in, 2 out]
        n280 = flat-sequence {
          tunnel: [w539] -> w364
          tunnel: [w518] -> w363
          tunnel: [w529] -> w362
          tunnel: [w509] -> w361
          tunnel: w350 -> [w508]
          tunnel: w349 -> [w507]
          tunnel: w364 -> [w543]
          tunnel: [w543] -> w360
          tunnel: w363 -> [w542]
          tunnel: [w542] -> w359
          tunnel: w362 -> [w541]
          tunnel: [w541] -> w358
          tunnel: w361 -> [w540]
          tunnel: [w540] -> w357
          tunnel: w360 -> [w546]
          tunnel: [w547] -> w356
          tunnel: w359 -> [w549]
          tunnel: [w548] -> w355
          tunnel: w358 -> [w545]
          tunnel: [w544] -> w354
          tunnel: w357 -> [w544]
          tunnel: w356 -> [w559]
          tunnel: w355 -> [w560]
          tunnel: w354 -> [w561]
          tunnel: [w558] -> w352
          tunnel: [w557] -> w353
          frame #0 {
            w513 = 0.1 ("Delay Time (s)")
            n281 = property on="Z Step SP" class="DigNum (strict)" props=["Maximum"]() -> ()  [unwired: 2 in, 3 out]
            n282 = call "mDrive Send Command.vi"("error in (no error)"=w507, "Extra"="P", "Command"=T1."Print Parameter", "VISA resource name"=w508) -> ("error out"=w534:errorcluster, "read buffer"=w538:string, "VISA resource name out"=w536:refnum<visa-resource-name>)  [unwired: 3 in]
            n283 = Decimal String To Number(string=w538, offset=0) -> (number=w520:i32)  [unwired: 1 in, 1 out]
            n284 = property on="Z Step SP" class="DigNum (strict)"() -> ("Minimum"=w532:dbl)  [unwired: 2 in, 2 out]
            n285 = property on="Z max step" class="DigNum (strict)"() -> ("Value"=w503:i32)  [unwired: 2 in, 2 out]
            n286 = To Long Integer(number=w520) -> (32bit integer=w521:i32)
            n287 = property on="Z Step PV" class="DigNum (strict)"("Val(Sgnl)"=w521) -> ()  [unwired: 2 in, 2 out]
            n288 = call "Time Delay17"("error in (no error)"=w534, "Delay Time (s)"=w513) -> ("error out"=w533:errorcluster)  [unwired: 9 in]
            n289 = To Long Integer(number=w532) -> (32bit integer=w531:i32)
            n290 = To Long Integer(number=w503) -> (32bit integer=w530:i32)
            n291 = property on="Z steps/rev" class="DigNum (strict)"() -> ("Value"=w527:u32)  [unwired: 2 in, 2 out]
            n292 = To Double Precision Float(number=w527) -> (double precision float=w528:dbl)
            n293 = In Range and Coerce(upper limit=w530, x=w521, lower limit=w531) -> (In Range?=w529:bool)  [unwired: 1 out]
            n294 = To Double Precision Float(number=w521) -> (double precision float=w522:dbl)
            n295 = Divide(x=w522, y=w528) -> (x/y=w526:dbl)
            n296 = property on="APX:MZ_LIM+" class="Bool (strict)"("Val(Sgnl)"=w529) -> ()  [unwired: 2 in, 2 out]
            n297 = call "mDrive Send Command.vi"("error in (no error)"=w533, "Extra"="MV", "Command"=T1."Print Parameter", "VISA resource name"=w536) -> ("error out"=w535:errorcluster, "read buffer"=w504:string, "VISA resource name out"=w539:refnum<visa-resource-name>)  [unwired: 3 in]
            n298 = call "Time Delay16"("error in (no error)"=w535, "Delay Time (s)"=w513) -> ("error out"=w518:errorcluster)  [unwired: 9 in]
            n299 = Decimal String To Number(string=w504, offset=0 ("offset (0)")) -> (number=w512:i32)  [unwired: 1 in, 1 out]
            n300 = Not Equal?(x=w504, y="") -> (x != y?=w505:bool)
            n301 = property on="Z mm/rev" class="DigNum (strict)"() -> ("Value"=w525:dbl)  [unwired: 2 in, 2 out]
            n302 = property on="Z offset mm" class="DigNum (strict)"() -> ("Value"=w523:dbl)  [unwired: 2 in, 2 out]
            n303 = Multiply(x=w526, y=w525) -> (x*y=w524:dbl)
            n304 = Number To Boolean Array(number=w512) -> (Boolean array=w511:bool[])
            n305 = property on="APX:MZ_RDY" class="Bool (strict)"("Val(Sgnl)"=w505) -> ()  [unwired: 2 in, 2 out]
            n306 = Add(x=w524, y=w523) -> (x+y=w502:dbl)
            n307 = Index Array(array=w511, index=0) -> (element=w509:bool)
            n308 = property on="APX:MZ_PV" class="DigNum (strict)"("Val(Sgnl)"=w502) -> ()  [unwired: 2 in, 2 out]
            n309 = property on="APX:MZ_MVG" class="Bool (strict)"("Val(Sgnl)"=w509) -> ()  [unwired: 2 in, 2 out]
          }
          frame #1 {
          }
          frame #2 {
            n310 = case shown="True" w545 {
              tunnel: w546 -> [w552 w556]
              tunnel: [w553 w556] -> w547
              tunnel: [w554 w555] -> w548
              tunnel: w549 -> [w551 w555]
              frame False {
                n311 = call "mDrive Send Command.vi"("error in (no error)"=w551, "Command"=T1."Stop", "VISA resource name"=w552) -> ("error out"=w554:errorcluster, "VISA resource name out"=w553:refnum<visa-resource-name>)  [unwired: 4 in, 1 out]
              }
              frame True {
              }
            }
          }
          frame #3 {
            n312 = disable-structure shown="Enabled" {
              disable-tunnel: w561 -> [w567 _]
              disable-tunnel: w560 -> [w565 _]
              disable-tunnel: w559 -> [w564 _]
              disable-tunnel: [w563 _] -> w558
              disable-tunnel: [w562 _] -> w557
              frame Disabled {
                n313 = Implies(1:w567) -> (0:w566:bool, 2:w568:bool)
                n314 = case shown="False" w566 {
                  tunnel: w565 -> [w575 w628]
                  tunnel: w564 -> [w574 w629]
                  tunnel: [w573 w628] -> w563
                  tunnel: [w572 w629] -> w562
                  frame False {
                    # "Backlash"
                    n315 = flat-sequence {
                      tunnel: [w590] -> w587
                      tunnel: [w592] -> w586
                      tunnel: [w591] -> w585
                      tunnel: w575 -> [w589]
                      tunnel: w574 -> [w588]
                      tunnel: w587 -> [w600]
                      tunnel: [w600] -> w584
                      tunnel: w586 -> [w599]
                      tunnel: w585 -> [w598]
                      tunnel: [w597] -> w583
                      tunnel: [w596] -> w582
                      tunnel: [w595] -> w571
                      tunnel: w584 -> [w610]
                      tunnel: w583 -> [w609]
                      tunnel: w582 -> [w607]
                      tunnel: [w608] -> w581
                      tunnel: [w607] -> w580
                      tunnel: [w606] -> w577
                      tunnel: [w605] -> w576
                      tunnel: w571 -> [w605]
                      tunnel: w581 -> [w621]
                      tunnel: w580 -> [w614]
                      tunnel: [w621] -> w579
                      tunnel: [w620] -> w578
                      tunnel: w577 -> [w620]
                      tunnel: w576 -> [w616]
                      tunnel: [w615] -> w569
                      tunnel: w579 -> [w625]
                      tunnel: w578 -> [w624]
                      tunnel: [w623] -> w573
                      tunnel: [w622] -> w570
                      tunnel: w569 -> [w622]
                      tunnel: [w627] -> w572
                      tunnel: w570 -> [w627]
                      frame #0 {
                        n316 = property on="Z Backlash steps/sec" class="DigNum (strict)"() -> ("Value"=w590:i32)  [unwired: 2 in, 2 out]
                        n317 = Number To Decimal String(number=w590) -> (decimal integer string=w593:string)  [unwired: 1 in]
                        n318 = call "mDrive Send Command.vi"("error in (no error)"=w589, "Extra"=w593, "Command"=T1."Max Velocity", "VISA resource name"=w588) -> ("error out"=w591:errorcluster, "VISA resource name out"=w592:refnum<visa-resource-name>)  [unwired: 3 in, 1 out]
                      }
                      frame #1 {
                        n319 = property on="Z Backlash" class="DigNum (strict)"() -> ("Value"=w595:i32)  [unwired: 2 in, 2 out]
                        n320 = Number To Decimal String(number=w595) -> (decimal integer string=w601:string)  [unwired: 1 in]
                        n321 = call "mDrive Send Command.vi"("error in (no error)"=w598, "Extra"=w601, "Command"=T1."Move to Relative Position", "VISA resource name"=w599) -> ("error out"=w597:errorcluster, "VISA resource name out"=w596:refnum<visa-resource-name>)  [unwired: 3 in, 1 out]
                      }
                      frame #2 {
                        n322 = To Double Precision Float(number=w605) -> (double precision float=w603:dbl)
                        n323 = To Double Precision Float(number=w610) -> (double precision float=w612:dbl)
                        n324 = Absolute Value(x=w603) -> (abs(x)=w604:dbl)
                        n325 = Divide(x=w604, y=w612) -> (x/y=w613:dbl)
                        n326 = Add(x=w613, y=0.5) -> (x+y=w606:dbl)
                        n327 = call "Time Delay18"("error in (no error)"=w609, "Delay Time (s)"=w606) -> ("error out"=w608:errorcluster)  [unwired: 9 in]
                      }
                      frame #3 {
                        n328 = Negate(x=w616) -> (-x=w617:i32)
                        n329 = Number To Decimal String(number=w617) -> (decimal integer string=w618:string)  [unwired: 1 in]
                        n330 = call "mDrive Send Command.vi"("Extra"=w618, "Command"=T1."Move to Relative Position", "VISA resource name"=w614) -> ("VISA resource name out"=w615:refnum<visa-resource-name>)  [unwired: 4 in, 2 out]
                      }
                      frame #4 {
                        n331 = call "Time Delay19"("error in (no error)"=w625, "Delay Time (s)"=w624) -> ("error out"=w623:errorcluster)  [unwired: 9 in]
                      }
                      frame #5 {
                        w626 = FALSE ("Value (Signaling)")
                      }
                    }
                  }
                  frame True {
                  }
                }
              }
              frame Enabled {
              }
            }
          }
        }
      }
      event "Reset Z Position mm": Value Change {
        n332 = event-data() -> ()  [unwired: 1 in, 5 out]
        n333 = property on="Reset Z Position mm" class="DigNum (strict)"() -> ("Value"=w638:dbl)  [unwired: 2 in, 2 out]
        n334 = property on="Z offset mm" class="DigNum (strict)"() -> ("Value"=w630:dbl)  [unwired: 2 in, 2 out]
        n335 = Subtract(x=w638, y=w630) -> (x-y=w637:dbl)
        n336 = property on="Z steps/rev" class="DigNum (strict)"() -> ("Value"=w632:u32)  [unwired: 2 in, 2 out]
        n337 = property on="Z mm/rev" class="DigNum (strict)"() -> ("Value"=w631:dbl)  [unwired: 2 in, 2 out]
        n338 = Divide(x=w637, y=w631) -> (x/y=w636:dbl)
        n339 = To Double Precision Float(number=w632) -> (double precision float=w635:dbl)
        n340 = Multiply(x=w636, y=w635) -> (x*y=w634:dbl)
        n341 = To Long Integer(number=w634) -> (32bit integer=w633:i32)
        n342 = property on="Reset Z Motor Steps" class="DigNum (strict)"("Val(Sgnl)"=w633) -> ()  [unwired: 2 in, 2 out]
      }
      event "Z Velocity SP step/sec", "Z Step SP": Value Change {
        n343 = event-data() -> ()  [unwired: 1 in, 5 out]
        n344 = property on="Z Velocity SP step/sec" class="DigNum (strict)"() -> ("Value"=w650:i32)  [unwired: 2 in, 2 out]
        n345 = property on="Z steps/rev" class="DigNum (strict)"() -> ("Value"=w641:u32)  [unwired: 2 in, 2 out]
        n346 = property on="Z steps/rev" class="DigNum (strict)"() -> ("Value"=w648:u32)  [unwired: 2 in, 2 out]
        n347 = property on="Z Step SP" class="DigNum (strict)"() -> ("Value"=w643:i32)  [unwired: 2 in, 2 out]
        n348 = To Double Precision Float(number=w643) -> (double precision float=w644:dbl)
        n349 = To Double Precision Float(number=w641) -> (double precision float=w647:dbl)
        n350 = To Double Precision Float(number=w650) -> (double precision float=w651:dbl)
        n351 = To Double Precision Float(number=w648) -> (double precision float=w653:dbl)
        n352 = Divide(x=w644, y=w647) -> (x/y=w646:dbl)
        n353 = Divide(x=w651, y=w653) -> (x/y=w652:dbl)
        n354 = property on="Z mm/rev" class="DigNum (strict)"() -> ("Value"=w639:dbl)  [unwired: 2 in, 2 out]
        n355 = property on="Z offset mm" class="DigNum (strict)"() -> ("Value"=w640:dbl)  [unwired: 2 in, 2 out]
        n356 = Multiply(x=w646, y=w639) -> (x*y=w645:dbl)
        n357 = Multiply(x=w652, y=w639) -> (x*y=w649:dbl)
        n358 = property on="APX:MZ_VLC_PV" class="DigNum (strict)"("Val(Sgnl)"=w649) -> ()  [unwired: 2 in, 2 out]
        n359 = Add(x=w645, y=w640) -> (x+y=w642:dbl)
        n360 = property on="Z Position MV mm" class="DigNum (strict)"("Val(Sgnl)"=w642) -> ()  [unwired: 2 in, 2 out]
      }
      event "APX:MZ_RQ": Value Change {
        n361 = event-data() -> ()  [unwired: 1 in, 6 out]
        n362 = property on="APX:MZ_RQ" class="DigNum (strict)"() -> ("Value"=w658:dbl)  [unwired: 2 in, 2 out]
        n363 = property on="APX:MZ_PV" class="DigNum (strict)"() -> ("Value"=w657:dbl)  [unwired: 2 in, 2 out]
        n364 = Less?(x=w658, y=w657) -> (x < y?=w654:bool)
        n365 = property on="Isolated from GND?" class="Bool (strict)"() -> ("Value"=w656:bool)  [unwired: 2 in, 2 out]
        n366 = Or(x=w656, y=w654) -> (x .or. y?=w655:bool)
        n367 = case shown="True" w655 {
          tunnel: w662 -> [w664 w668]
          tunnel: w661 -> [w663 w667]
          tunnel: [w663 w666] -> w660
          tunnel: [w664 w665] -> w659
          frame False {
          }
          frame True {
            n368 = flat-sequence {
              tunnel: w667 -> [w677]
              tunnel: w668 -> [w678]
              tunnel: [w678] -> w676
              tunnel: [w677] -> w675
              tunnel: [w700] -> w674
              tunnel: [w699] -> w673
              tunnel: w676 -> [w702]
              tunnel: w675 -> [w701]
              tunnel: [w718] -> w672
              tunnel: [w717] -> w671
              tunnel: w674 -> [w716]
              tunnel: w673 -> [w715]
              tunnel: [w726] -> w670
              tunnel: [w725] -> w669
              tunnel: w672 -> [w724]
              tunnel: w671 -> [w723]
              tunnel: [w732] -> w666
              tunnel: [w733] -> w665
              tunnel: w670 -> [w733]
              tunnel: w669 -> [w731]
              frame #0 {
                (unwired) T2."Disabled and Grayed Out" ("Disabled")
                (unwired) T2."Disabled and Grayed Out" ("Disabled")
                n369 = flat-sequence {
                  frame #0 {
                    n370 = property on="APX:MZ_RQ" class="DigNum (strict)"() -> ("Value"=w690:dbl)  [unwired: 2 in, 2 out]
                    n371 = property on="Z offset mm" class="DigNum (strict)"() -> ("Value"=w691:dbl)  [unwired: 2 in, 2 out]
                    n372 = property on="APX:MZ_VLC_RQ" class="DigNum (strict)"() -> ("Value"=w684:dbl)  [unwired: 2 in, 2 out]
                    n373 = property on="Z steps/rev" class="DigNum (strict)"() -> ("Value"=w693:u32)  [unwired: 2 in, 2 out]
                    n374 = property on="Z mm/rev" class="DigNum (strict)"() -> ("Value"=w696:dbl)  [unwired: 2 in, 2 out]
                    n375 = Subtract(x=w690, y=w691) -> (x-y=w694:dbl)
                    n376 = property on="Z Velocity SP step/sec" class="DigNum (strict)"() -> ("Maximum"=w680:dbl)  [unwired: 2 in, 2 out]
                    n377 = property on="Z Velocity SP step/sec" class="DigNum (strict)"() -> ("Minimum"=w679:dbl)  [unwired: 2 in, 2 out]
                    n378 = Divide(x=w684, y=w696) -> (x/y=w685:dbl)
                    n379 = Divide(x=w694, y=w696) -> (x/y=w695:dbl)
                    n380 = To Double Precision Float(number=w693) -> (double precision float=w697:dbl)
                    n381 = property on="Z Step SP" class="DigNum (strict)"() -> ("Maximum"=w687:dbl)  [unwired: 2 in, 2 out]
                    n382 = property on="Z Step SP" class="DigNum (strict)"() -> ("Minimum"=w686:dbl)  [unwired: 2 in, 2 out]
                    n383 = Multiply(x=w685, y=w697) -> (x*y=w682:dbl)
                    n384 = Multiply(x=w695, y=w697) -> (x*y=w689:dbl)
                    n385 = In Range and Coerce(upper limit=w680, x=w682, lower limit=w679) -> (coerced(x)=w681:dbl)  [unwired: 1 out]
                    n386 = In Range and Coerce(upper limit=w687, x=w689, lower limit=w686) -> (coerced(x)=w688:dbl)  [unwired: 1 out]
                    n387 = To Long Integer(number=w681) -> (32bit integer=w683:i32)
                    n388 = To Long Integer(number=w688) -> (32bit integer=w692:i32)
                    n389 = property on="Z Velocity SP step/sec" class="DigNum (strict)"("Val(Sgnl)"=w683) -> ()  [unwired: 2 in, 2 out]
                    n390 = property on="Z Step SP" class="DigNum (strict)"("Val(Sgnl)"=w692) -> ()  [unwired: 2 in, 2 out]
                  }
                }
              }
              frame #1 {
                n391 = property on="Z Step SP" class="DigNum (strict)"() -> ("Value"=w710:i32)  [unwired: 2 in, 2 out]
                n392 = property on="Z Step PV" class="DigNum (strict)"() -> ("Value"=w709:i32)  [unwired: 2 in, 2 out]
                n393 = property on="Z Backlash" class="DigNum (strict)"() -> ("Value"=w698:i32)  [unwired: 2 in, 2 out]
                n394 = Subtract(x=w710, y=w709) -> (x-y=w708:i32)
                n395 = Sign(1:w708) -> (0:w707:i32)
                n396 = Sign(1:w698) -> (0:w706:i32)
                n397 = Multiply(x=w707, y=w706) -> (x*y=w705:i32)
                n398 = Equal?(x=w705, y=1) -> (x = y?=w703:bool)
                n399 = case shown="True" w703 {
                  tunnel: w702 -> [w712 w714]
                  tunnel: w701 -> [w711 w713]
                  tunnel: [w711 w713] -> w700
                  tunnel: [w712 w714] -> w699
                  frame False {
                    (unwired) FALSE ("Value (Signaling)")
                  }
                  frame True {
                    (unwired) TRUE ("Value (Signaling)")
                  }
                }
              }
              frame #2 {
                # "Velocity Setting"
                n400 = property on="Z Velocity SP step/sec" class="DigNum (strict)"() -> ("Value"=w719:i32)  [unwired: 2 in, 2 out]
                n401 = Number To Decimal String(number=w719) -> (decimal integer string=w720:string)  [unwired: 1 in]
                n402 = call "mDrive Send Command.vi"("error in (no error)"=w716, "Extra"=w720, "Command"=T1."Max Velocity", "VISA resource name"=w715) -> ("error out"=w717:errorcluster, "VISA resource name out"=w718:refnum<visa-resource-name>)  [unwired: 3 in, 1 out]
              }
              frame #3 {
                # "Move to Abs Position"
                n403 = call "Time Delay7"("error in (no error)"=w723) -> ("error out"=w722:errorcluster)  [unwired: 10 in]
                n404 = property on="Z Step SP" class="DigNum (strict)"() -> ("Value"=w729:i32)  [unwired: 2 in, 2 out]
                n405 = Number To Decimal String(number=w729) -> (decimal integer string=w728:string)  [unwired: 1 in]
                n406 = call "mDrive Send Command.vi"("error in (no error)"=w722, "Extra"=w728, "Command"=T1."Move to Absolute Position", "VISA resource name"=w724) -> ("error out"=w725:errorcluster, "VISA resource name out"=w726:refnum<visa-resource-name>)  [unwired: 3 in, 1 out]
              }
              frame #4 {
                n407 = call "Time Delay28"("error in (no error)"=w731, "Delay Time (s)"=0.1) -> ("error out"=w732:errorcluster)  [unwired: 9 in]
              }
            }
          }
        }
      }
      event "APX:MZ_STOP_Button": Mouse Down {
        n408 = flat-sequence {
          tunnel: [w741] -> w735
          tunnel: [w740] -> w734
          tunnel: w737 -> [w739]
          tunnel: w736 -> [w738]
          frame #0 {
            n409 = call "mDrive Send Command.vi"("error in (no error)"=w738, "Command"=T1."Stop", "VISA resource name"=w739) -> ("error out"=w740:errorcluster, "VISA resource name out"=w741:refnum<visa-resource-name>)  [unwired: 4 in, 1 out]
          }
        }
        n410 = event-data() -> ()  [unwired: 1 in, 8 out]
      }
      event "Reset": Mouse Down {
        n411 = flat-sequence {
          frame #0 {
          }
        }
        n412 = flat-sequence {
          frame #0 {
          }
        }
        n413 = event-data() -> ()  [unwired: 1 in, 7 out]
        n414 = flat-sequence {
          frame #0 {
          }
        }
        n415 = flat-sequence {
          tunnel: [w750] -> w744
          tunnel: [w749] -> w743
          tunnel: w746 -> [w748]
          tunnel: w745 -> [w747]
          frame #0 {
            n416 = property on="Reset Z Motor Steps" class="DigNum (strict)"() -> ("Value"=w751:i32)  [unwired: 2 in, 2 out]
            n417 = Number To Decimal String(number=w751) -> (decimal integer string=w752:string)  [unwired: 1 in]
            n418 = call "mDrive Send Command.vi"("error in (no error)"=w747, "Extra"=w752, "Command"=T1."Set Current Position", "VISA resource name"=w748) -> ("error out"=w749:errorcluster, "VISA resource name out"=w750:refnum<visa-resource-name>)  [unwired: 3 in, 1 out]
          }
        }
      }
    }
  }
  n419 = flat-sequence {
    tunnel: w21 -> [w760]
    tunnel: w20 -> [w758]
    tunnel: [w755] -> w19
    frame #0 {
      n420 = call "mDrive Send Command.vi"("error in (no error)"=w758, "Extra"="P", "Command"=T1."Print Parameter", "VISA resource name"=w760) -> ("error out"=w757:errorcluster, "read buffer"=w764:string, "VISA resource name out"=w759:refnum<visa-resource-name>)  [unwired: 3 in]
      n421 = call "Time Delay32"("error in (no error)"=w757) -> ("error out"=w754:errorcluster)  [unwired: 10 in]
      n422 = Decimal String To Number(string=w764, offset=0) -> (number=w756:i32)  [unwired: 1 in, 1 out]
      n423 = To Long Integer(number=w756) -> (32bit integer=w755:i32)
      n424 = call "mDrive Send Command.vi"("error in (no error)"=w754, "Command"=T1."Stop", "VISA resource name"=w759) -> ("error out"=w766:errorcluster, "VISA resource name out"=w767:refnum<visa-resource-name>)  [unwired: 4 in, 1 out]
      n425 = VISA Close(VISA resource name=w767, error in (no error)=w766) -> ()  [unwired: 1 out]
    }
  }
  n426 = flat-sequence {
    tunnel: w19 -> [w773]
    frame #0 {
      n427 = Build Array(0 ("element"), 0 ("element"), w773, 0 ("element")) -> (w771:i32[])
      n428 = call-poly <vilib>:"Write To Spreadsheet File.vi"("1D data"=w771, "file path (dialog if empty)"=path "T:/PAR/IMS/POSZ.TXT") -> ()  [unwired: 6 in, 1 out]
    }
    frame #1 {
    }
  }
